vi "3 Tap 8-Bit.vi"() -> (0 "Pixels":T1)   [LabVIEW 2015]
uses:
  <vilib>/rvi/eio/common/nirviEmuTemplateMethod_errors.vi
  <vilib>/eio/EIONode/EIONode.xnode
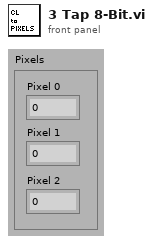
[diagram p1: front panel]
types:
  T1 = cluster{"Pixel 0":u8, "Pixel 1":u8, "Pixel 2":u8}
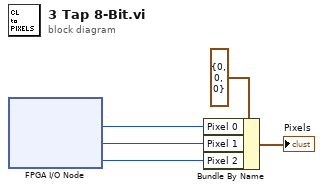
[diagram p0: block diagram]
diagram:
  n1 = xnode "FPGA I/O Node"() -> ("CL Port A"=w5:u8, "CL Port B"=w4:u8, "CL Port C"=w1:u8)  [unwired: 3 in, 3 out]
  n2 = Bundle By Name(cluster=T1 {"Pixel 0"=0, "Pixel 1"=0, "Pixel 2"=0} ("PixelData"), "Pixel 0"=w5, "Pixel 1"=w4, "Pixel 2"=w1) -> (→"Pixels":T1)
